vi "Write String.vi"(7 "Channel Name":string, 8 "error in (no error)":errorcluster, 9 "Data Value":dbl, 10 "Bus In":refnum<class "Bus.lvclass">, 11 "No-Op in":refnum<class "No-Op Channel.lvclass">) -> (0 "error out":errorcluster, 2 "Bus Out":refnum<class "Bus.lvclass">, 3 "No-Op out":refnum<class "No-Op Channel.lvclass">)   [LabVIEW 2018, in "No-Op Channel.lvclass"]
doc: "String Out.lvclass:Read String.vi\n\nThis is the template for the Read String VI forthe String Out class.\n\nInstrument Communication Module Version 1.0\nOctober, 2020 Original Code Consulting Davita Bird\n www.originalcode.com"
uses:
  No-Op Channel.lvclass
  Bus/Bus.lvclass
  No-Op Channel.lvclass/No-Op Channel.ctl
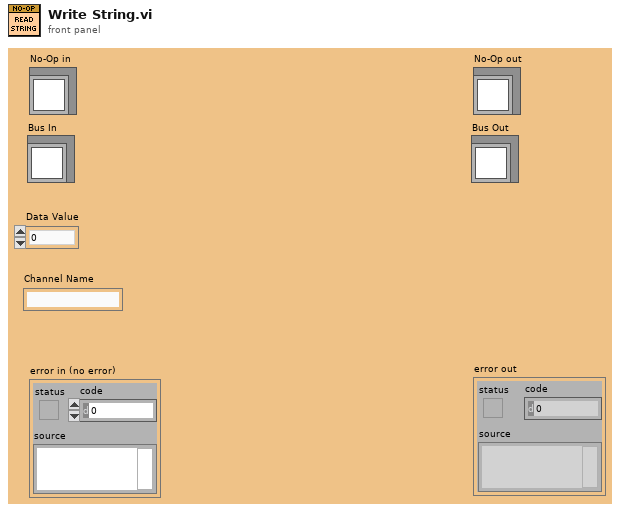
[diagram p1: front panel]
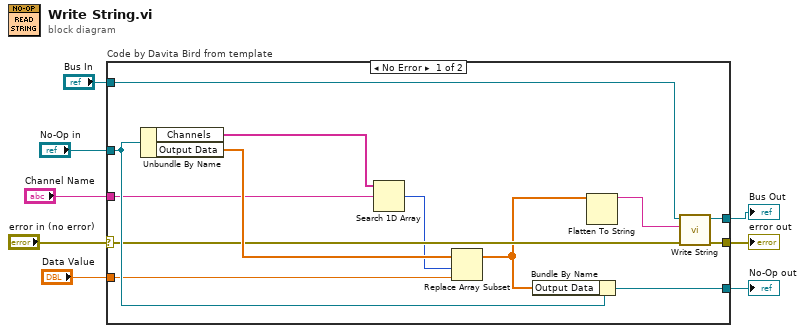
[diagram p0: block diagram]
diagram:
  n1 = case "Code by Davita Bird from template" shown="No Error" "error in (no error)" {
    selector: "error in (no error)" -> [w14 w24]
    tunnel: [w18 w24] -> w7
    tunnel: [w17 w23] -> w6
    tunnel: "No-Op in" -> [w21 w23]
    tunnel: "Data Value" -> [w15 _]
    tunnel: "Bus In" -> [w19 w22]
    tunnel: [w20 w22] -> w3
    tunnel: "Channel Name" -> [w11 _]
    frame No Error {
      n2 = Unbundle By Name(w21) -> ("Channels"=w9:string[], "Output Data"=w16:dbl[])
      n3 = Search 1D Array(1D array=w9, element=w11) -> (index of element=w10:i32)  [unwired: 1 in]
      n4 = Replace Array Subset(array=w16, new element=w15, index=w10) -> (w12:dbl[])
      n5 = Bundle By Name(cluster=w21, "Output Data"=w12) -> (w17:refnum<class "No-Op Channel.lvclass">)
      n6 = Flatten To String(anything=w12) -> (data string=w13:string)  [unwired: 3 in, 2 out]
      n7 = call-dynamic "Write String.vi"("error in (no error)"=w14, "String"=w13, "Bus in"=w19) -> ("error out"=w18:errorcluster, "Bus out"=w20:refnum<class "Bus.lvclass">)  [unwired: 7 in]
    }
    frame Error {
    }
  }
  "error out" <- w7
  "No-Op out" <- w6
  "Bus Out" <- w3
